vi "Configure Trigger.vi"(8 "error in (no error)":errorcluster, 9 "trigger delay (sec)":dbl format="%.3f", 10 "trigger source (int:0)":u16(ring) items=["internal", "external", "manual", "bus"], 11 "VISA resource name":refnum<visa-resource-name>) -> (0 "error out":errorcluster, 3 "VISA resource name out":refnum<visa-resource-name>)   [LabVIEW 2016, in "Agilent 4263X.lvlib"]
doc: "This VI configures the trigger mode and trigger delay."
uses:
  <instrlib>/Agilent 4263X/Agilent 4263X.lvlib
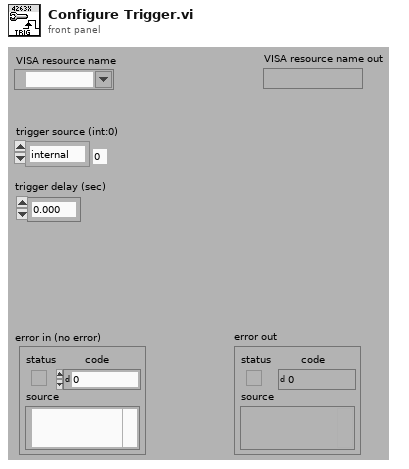
[diagram p1: front panel]
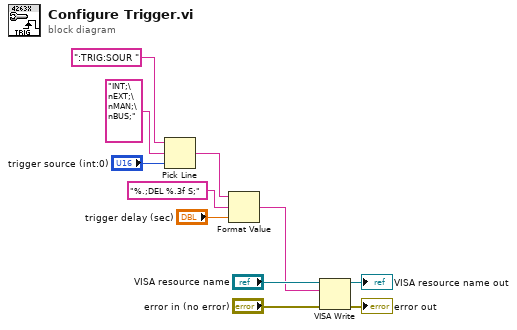
[diagram p0: block diagram]
diagram:
  n1 = Pick Line(string ("")=":TRIG:SOUR ", multi-line string="INT;\nEXT;\nMAN;\nBUS;", line index="trigger source (int:0)") -> (output string=w4:string)
  n2 = Format Value(string ("")=w4, format string="%.;DEL %.3f S;", value (0)="trigger delay (sec)") -> (output string=w1:string)
  n3 = VISA Write(VISA resource name="VISA resource name", write buffer=w1, error in (no error)="error in (no error)") -> (VISA resource name out=→"VISA resource name out":refnum<visa-resource-name>, error out=→"error out":errorcluster)  [unwired: 1 out]
